vi "Select Categories Like Name.vi"(8 "error in (no error)":errorcluster, 10 "Name filter":string, 11 "Database in":refnum<class "Database.lvclass">) -> (0 "error out":errorcluster, 2 "Categories":refnum<class "Category.lvclass">[](array[class]), 3 "Database out":refnum<class "Database.lvclass">)   [LabVIEW 2018, in "Database.lvclass"]
uses:
  Database.lvclass
  Category/Category.lvclass
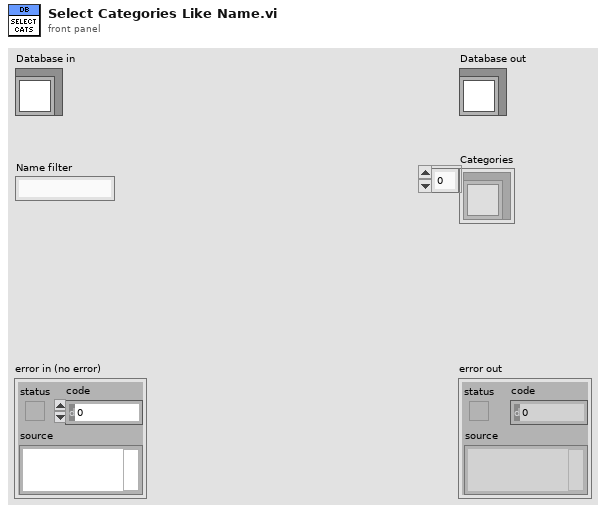
[diagram p1: front panel]
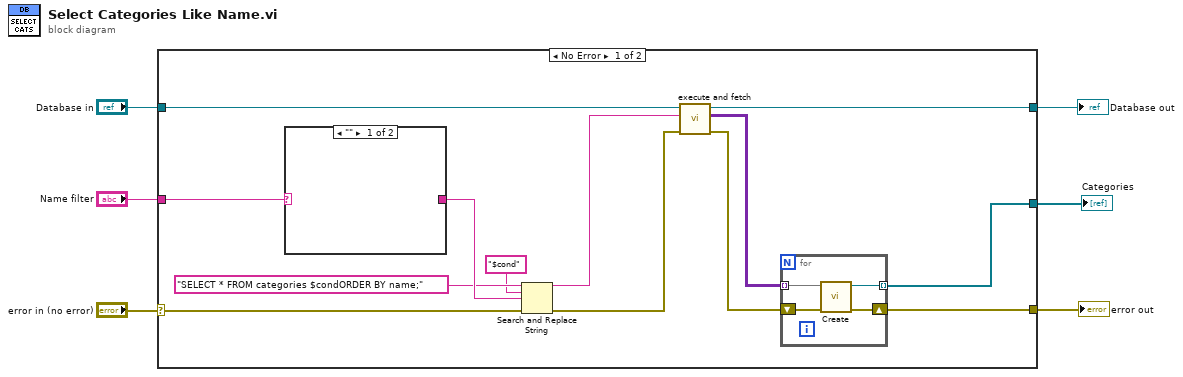
[diagram p0: block diagram]
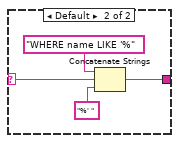
[diagram p2: hidden frame]
diagram:
  n1 = case shown="No Error" "error in (no error)" {
    selector: "error in (no error)" -> [w7 w28]
    tunnel: [w12 w29] -> w6
    tunnel: "Database in" -> [w11 w29]
    tunnel: [w10 w28] -> w4
    tunnel: "Name filter" -> [w9 _]
    tunnel: [w8 _] -> w2
    frame No Error {
      n2 = case shown="\"\"" w9 {
        selector: w9 -> [_ w20]
        tunnel: [_ w23] -> w16
        frame "" {
        }
        frame Default {
          n3 = Concatenate Strings("WHERE name LIKE '%", w20, "%' ") -> (w23:string)
        }
      }
      n4 = Search and Replace String(input string="SELECT * FROM categories $condORDER BY name;", search string="$cond", replace string=w16, error in=w7) -> (result string=w13:string, error out=w17:errorcluster)  [unwired: 4 in, 2 out]
      n5 = call "execute and fetch.vi"("error in (no error)"=w17, "SQL query"=w13, "Database in"=w11) -> ("error out"=w18:errorcluster, "recordset data"=w19:variant[][], "Database out"=w12:refnum<class "Database.lvclass">)  [unwired: 5 in, 1 out]
      n6 = for {
        tunnel: w19 -> [w27] mode=indexing
        shift-right: [w24] -> w10
        shift-left: w18 -> [w26]
        tunnel: [w25] -> w8 mode=indexing
        n7 = call "Create.vi"("error in (no error)"=w26, "Record"=w27) -> ("error out"=w24:errorcluster, "Category out"=w25:refnum<class "Category.lvclass">)  [unwired: 8 in]
      }
    }
    frame Error {
    }
  }
  "error out" <- w4
  "Database out" <- w6
  "Categories" <- w2
